vi "Update Chnls with DeActivateHW.vi"(8 "error in (no error)":errorcluster, 10 "ChnlSettings":T1[](array[typedef]) {"ChnParameter"."Delay (µs)" min=0.0 max=100000000.0 format="%.4f"; "G08_Chnl_Settings"."Pulse Width (µs)" min=0.0 max=8947840.0 format="%#.6f"; "Go and Done Signal"."Done Signal" format="%04x" items=["Local Primary"=1, "Local Secondary"=2, "Local Force"=4, "Master Primary"=16]; "Go and Done Signal"."Go Signal" format="%04x" items=["Local Primary0x1"=1, "Local Secondary0x2"=2, "Local Force 0x4"=4, "Resynchronize 0x8"=8, "Master Prim. 0x10"=16, "Master Sec. 0x20"=32, "Master Force  0x40"=64, "System Clock 0x80"=128, "Delay Clock 0x100"=256, "Inhibit Local 0x200"=512, "Start Local 0x400"=1024, "Start Bus 0x800"=2048, "Step Back Local 0x1000"=4096, "Step Back Bus 0x2000"=8192, "RunCircle 0x4000"=16384, "SyncReload 0x8000"=32768, "From E 0x10000"=65536, "From F 0x20000"=131072, "From Bus 0x40000"=262144]}, 11 "BME_DG_System in":refnum<class "BME_DG_System.lvclass">) -> (0 "error out":errorcluster, 2 "ProblemChnls":string[](array[string]), 3 "BME_DG_System out":refnum<class "BME_DG_System.lvclass">)   [LabVIEW 2009, in "POLARIS BME DG.lvlib" / "BME_DG_System.lvclass"]
uses:
  BME_DG_System.lvclass
  Chnl Settings Complete.ctl
  LV-BME Interface/ChnlSettings.ctl
  Go_Done_Chnl_Settings.ctl
  GoSignalBits.ctl
  SG08_Chnl_Settings.ctl
  BME_DG_Chnl/BME_DG_Chnl.lvclass
  POLARIS BME DG.lvlib
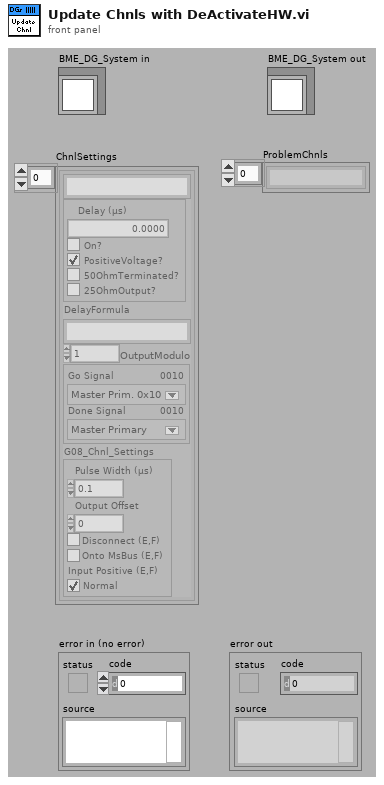
[diagram p1: front panel]
types:
  T1 = typedef "POLARIS BME DG.lvlib/Chnl Settings Complete.ctl" = cluster{"Channel Name":string, "ChnParameter":T2, "DelayFormula":string, "OutputModulo":i32, "Go and Done Signal":T3, "G08_Chnl_Settings":T5}
  T2 = typedef "POLARIS BME DG.lvlib/ChnlSettings.ctl" = cluster{" Delay (µs)":dbl, "On?":bool, "PositiveVoltage?":bool, "50OhmTerminated? ":bool, "25OhmOutput?":bool}
  T3 = typedef "POLARIS BME DG.lvlib/Go_Done_Chnl_Settings.ctl" = cluster{"Go Signal":T4, "Done Signal":u32}
  T4 = typedef "POLARIS BME DG.lvlib/GoSignalBits.ctl" = u32
  T5 = typedef "POLARIS BME DG.lvlib/SG08_Chnl_Settings.ctl" = cluster{"Pulse Width (µs)":dbl, "Output Offset":u32, "Disconnect (E,F)":bool, "Onto MsBus (E,F)":bool, "Input Positive (E,F)":bool}
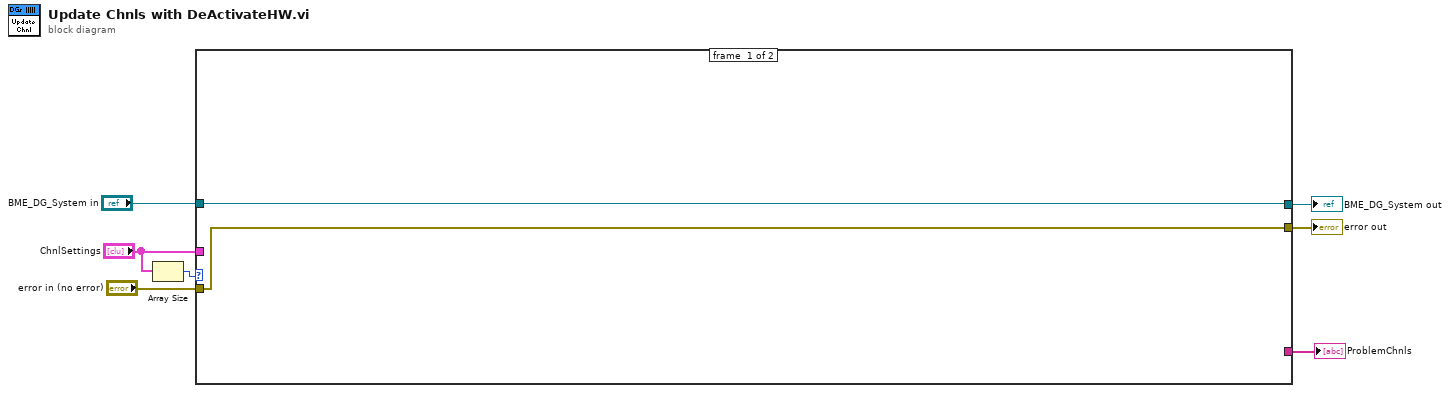
[diagram p0: block diagram]
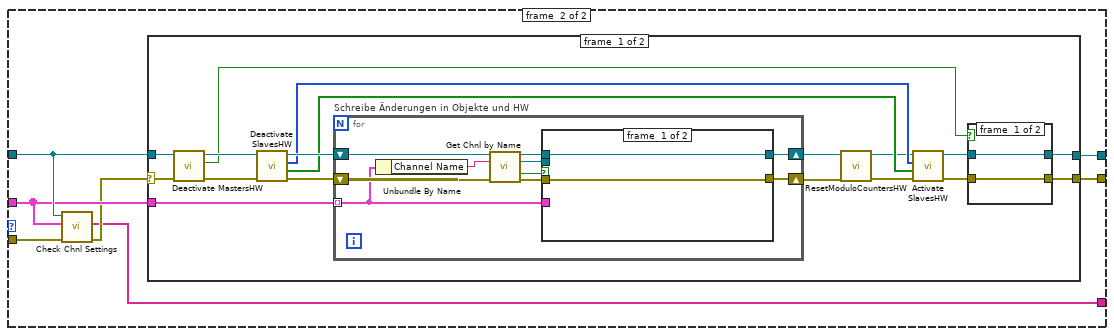
[diagram p2: hidden frame]
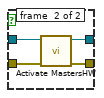
[diagram p3: hidden frame]
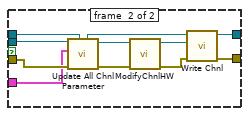
[diagram p4: hidden frame]
diagram:
  n1 = Array Size(array="ChnlSettings") -> (size(s)=w3:i32)
  n2 = case shown="1, Default" w3 {
    tunnel: [w8 w16] -> w7
    tunnel: [w9 w15] -> w6
    tunnel: "BME_DG_System in" -> [w9 w14]
    tunnel: "error in (no error)" -> [w8 w13]
    tunnel: "ChnlSettings" -> [_ w12]
    tunnel: [_ w10] -> w1
    frame #0 {
    }
    frame #1 {
      n3 = call "Check Chnl Settings.vi"("error in (no error)"=w13, "ChnlSettings"=w12, "BME_DG_System in"=w14) -> ("error out"=w11:errorcluster, "Problem Chnls out"=w10:string[])  [unwired: 7 in]
      n4 = case shown="No Error" w11 {
        selector: w11 -> [w30 w65]
        tunnel: [w22 w65] -> w16
        tunnel: [w23 w64] -> w15
        tunnel: w14 -> [w31 w64]
        tunnel: w12 -> [w34 _]
        frame #0 {
          n5 = call "Deactivate MastersHW.vi"("error in (no error)"=w30, "BME_DG_System in"=w31) -> ("error out"=w28:errorcluster, "Deactivated?"=w21:bool, "BME_DG_System out"=w29:refnum<class "BME_DG_System.lvclass">)  [unwired: 7 in]
          n6 = call "Deactivate SlavesHW.vi"("error in (no error)"=w28, "BME_DG_System in"=w29) -> ("error out"=w33:errorcluster, "has been deactivated?"=w25:bool[], "DGNrs"=w26:i32[], "BME_DG_System out"=w32:refnum<class "BME_DG_System.lvclass">)  [unwired: 6 in]
          n7 = for "Schreibe Änderungen in Objekte und HW" {
            shift-right: [w45] -> w20
            shift-left: w32 -> [w46]
            tunnel: w34 -> [w41] mode=indexing
            shift-right: [w42] -> w17
            shift-left: w33 -> [w43]
            n8 = Unbundle By Name(w41) -> ("Channel Name"=w44:string)
            n9 = call "Get Chnl by Name.vi"("BME_DG_System in"=w46, "Chnl Name"=w44, "error in (no error)"=w43) -> ("BME_DG_System out"=w48:refnum<class "BME_DG_System.lvclass">, "BME_DG_Chnl"=w49:refnum<class "BME_DG_Chnl.lvclass">, "found?"=w50:bool, "error out"=w47:errorcluster)  [unwired: 7 in, 2 out]
            n10 = case shown="True" w50 {
              tunnel: w49 -> [_ w60]
              tunnel: w48 -> [w52 w58]
              tunnel: w47 -> [w51 w61]
              tunnel: [w52 w62] -> w45
              tunnel: [w51 w63] -> w42
              tunnel: w41 -> [_ w59]
              frame #0 {
              }
              frame #1 {
                n11 = call "Update All Chnl Parameter.vi"("BME_DG_System in"=w58, "error in (no error)"=w61, "ChnlSettings"=w59, "BME_DG_Chnl in"=w60) -> ("error out"=w54:errorcluster, "BME_DG_Chnl out"=w56:refnum<class "BME_DG_Chnl.lvclass">, "BME_DG_System out"=w57:refnum<class "BME_DG_System.lvclass">)  [unwired: 5 in]
                n12 = call-dynamic "ModifyChnlHW.vi"("error in (no error)"=w54, "BME_DG_Chnl in"=w56) -> ("error out"=w53:errorcluster, "BME_DG_Chnl out"=w55:refnum<class "BME_DG_Chnl.lvclass">)  [unwired: 8 in]
                n13 = call "Write Chnl.vi"("error in (no error)"=w53, "BME_DG_Chnl.lvclass"=w55, "BME_DG_System in"=w57) -> ("error out"=w63:errorcluster, "BME_DG_System out"=w62:refnum<class "BME_DG_System.lvclass">)  [unwired: 7 in]
              }
            }
          }
          n14 = call "ResetModuloCountersHW.vi"("error in (no error)"=w17, "BME_DG_System in"=w20) -> ("error out"=w18:errorcluster, "BME_DG_System out"=w19:refnum<class "BME_DG_System.lvclass">)  [unwired: 8 in]
          n15 = call "Activate SlavesHW.vi"("error in (no error)"=w18, "has been deactivated?"=w25, "DGNrs"=w26, "BME_DG_System in"=w19) -> ("error out"=w24:errorcluster, "BME_DG_System out"=w27:refnum<class "BME_DG_System.lvclass">)  [unwired: 6 in]
          n16 = case shown="True" w21 {
            tunnel: w27 -> [w36 w40]
            tunnel: w24 -> [w35 w39]
            tunnel: [w36 w38] -> w23
            tunnel: [w35 w37] -> w22
            frame #0 {
            }
            frame #1 {
              n17 = call "Activate MastersHW.vi"("error in (no error)"=w39, "BME_DG_System in"=w40) -> ("error out"=w37:errorcluster, "BME_DG_System out"=w38:refnum<class "BME_DG_System.lvclass">)  [unwired: 8 in]
            }
          }
        }
        frame #1 {
        }
      }
    }
  }
  "error out" <- w7
  "BME_DG_System out" <- w6
  "ProblemChnls" <- w1
